vi "ScaleRectangeData.vi"(2 "X-In":sgl, 3 "Y-In":sgl, 4 "Width-In":sgl, 5 "Height-In":sgl, 6 "Offset(raw)":cluster{"x":sgl, "y":sgl}, 10 "Scale":dbl) -> (16 "X-Out":sgl, 17 "Y-Out":sgl, 18 "Width-Out":sgl, 19 "Height-Out":sgl)   [LabVIEW 2020, in "LcPictureBox.lvclass"]
uses:
  <userlib>/_LabVIEWCommon/LcPictureBox_class/LcPictureBox.lvclass
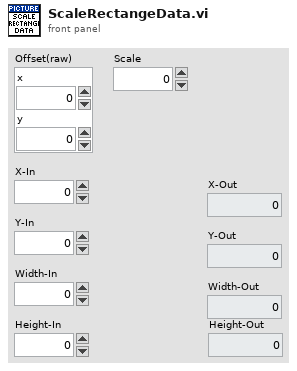
[diagram p1: front panel]
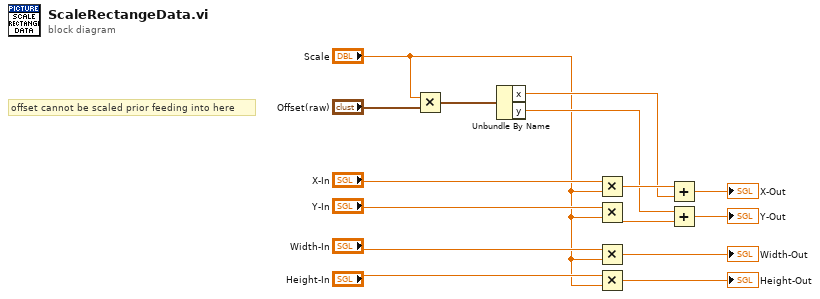
[diagram p0: block diagram]
diagram:
  # "offset cannot be scaled prior feeding into here"
  n1 = Multiply(x="Scale", y="Offset(raw)") -> (x*y=w1:cluster{"x":dbl, "y":dbl})
  n2 = Unbundle By Name(w1) -> ("x"=w10:dbl, "y"=w9:dbl)
  n3 = Multiply(x="X-In", y="Scale") -> (x*y=w11:dbl)
  n4 = Multiply(x="Y-In", y="Scale") -> (x*y=w8:dbl)
  n5 = Multiply(x="Width-In", y="Scale") -> (x*y=→"Width-Out":dbl)
  n6 = Multiply(x="Height-In", y="Scale") -> (x*y=→"Height-Out":dbl)
  n7 = Add(x=w11, y=w10) -> (x+y=→"X-Out":dbl)
  n8 = Add(x=w9, y=w8) -> (x+y=→"Y-Out":dbl)
